vi "Initialization.vi"(8 "error in":errorcluster, 11 "Data Cluster":T1={"Status"="", "Image"=[], "Device Settings"={"ROI"={"_Horizontal"=0, "_Horizontal Width"=0, "_Horizontal Binning"=0, "_Vertical"=0, "_Vertical Width"=0, "_Vertical Binning"=0}, "Gating"={"_GatingMode"=enum."None", "_RepetitiveGate"={"delay"=0.0, "width"=0.0}}, "Readout Control"={"Accumulations"=0}, "AD Conversion"={"AdcSpeed"=0.0, "AdcEMGain"=0, "AdcBitDepth"=0, "AdcAnalogGain"=enum."Low", "AdcQuality"=enum."LowNoise"}, "Intensifier"={"EnableIntensifier"=FALSE, "IntensifierStatus"=enum."None", "IntensifierGain"=0, "_EMIccdGainControlMode"=enum."None", "EMIccdGain"=0, "GatingSpeed"=enum."None"}, "Sensor Temperature"={"SensorTemperatureSetPoint"=0.0, "SensorTemperatureReading"=0.0, "SensorTemperatureStatus"=enum."None"}}, "-Picam Object"=refnum}) -> (0 "error out":errorcluster, 3 "Data Cluster out":T1={"Status"="", "Image"=[], "Device Settings"={"ROI"={"_Horizontal"=0, "_Horizontal Width"=0, "_Horizontal Binning"=0, "_Vertical"=0, "_Vertical Width"=0, "_Vertical Binning"=0}, "Gating"={"_GatingMode"=enum."None", "_RepetitiveGate"={"delay"=0.0, "width"=0.0}}, "Readout Control"={"Accumulations"=0}, "AD Conversion"={"AdcSpeed"=0.0, "AdcEMGain"=0, "AdcBitDepth"=0, "AdcAnalogGain"=enum."Low", "AdcQuality"=enum."LowNoise"}, "Intensifier"={"EnableIntensifier"=FALSE, "IntensifierStatus"=enum."None", "IntensifierGain"=0, "_EMIccdGainControlMode"=enum."None", "EMIccdGain"=0, "GatingSpeed"=enum."None"}, "Sensor Temperature"={"SensorTemperatureSetPoint"=0.0, "SensorTemperatureReading"=0.0, "SensorTemperatureStatus"=enum."None"}}, "-Picam Object"=refnum})   [LabVIEW 2019, in "Camera.lvlib"]
uses:
  Camera.lvlib
  Module Data--cluster.ctl
  Camera-LVClass/Picam_class/Picam.lvclass
  ROI--cluster.ctl
  picam32_LabView_SDK/PICam_lib/types/PicamGatingMode.ctl
  picam32_LabView_SDK/PICam_lib/types/PicamPulse.ctl
  picam32_LabView_SDK/PICam_lib/Ctrls/PicamAdcAnalogGain.ctl
  picam32_LabView_SDK/PICam_lib/Ctrls/PicamAdcQuality.ctl
  picam32_LabView_SDK/PICam_lib/types/PicamIntensifierStatus.ctl
  picam32_LabView_SDK/PICam_lib/types/PicamEMIccdGainControlMode.ctl
  picam32_LabView_SDK/PICam_lib/types/PicamGatingSpeed.ctl
  picam32_LabView_SDK/PICam_lib/types/PicamSensorTemperatureStatus.ctl
  picam32_LabView_SDK/PICam_lib/PICam.lvlib
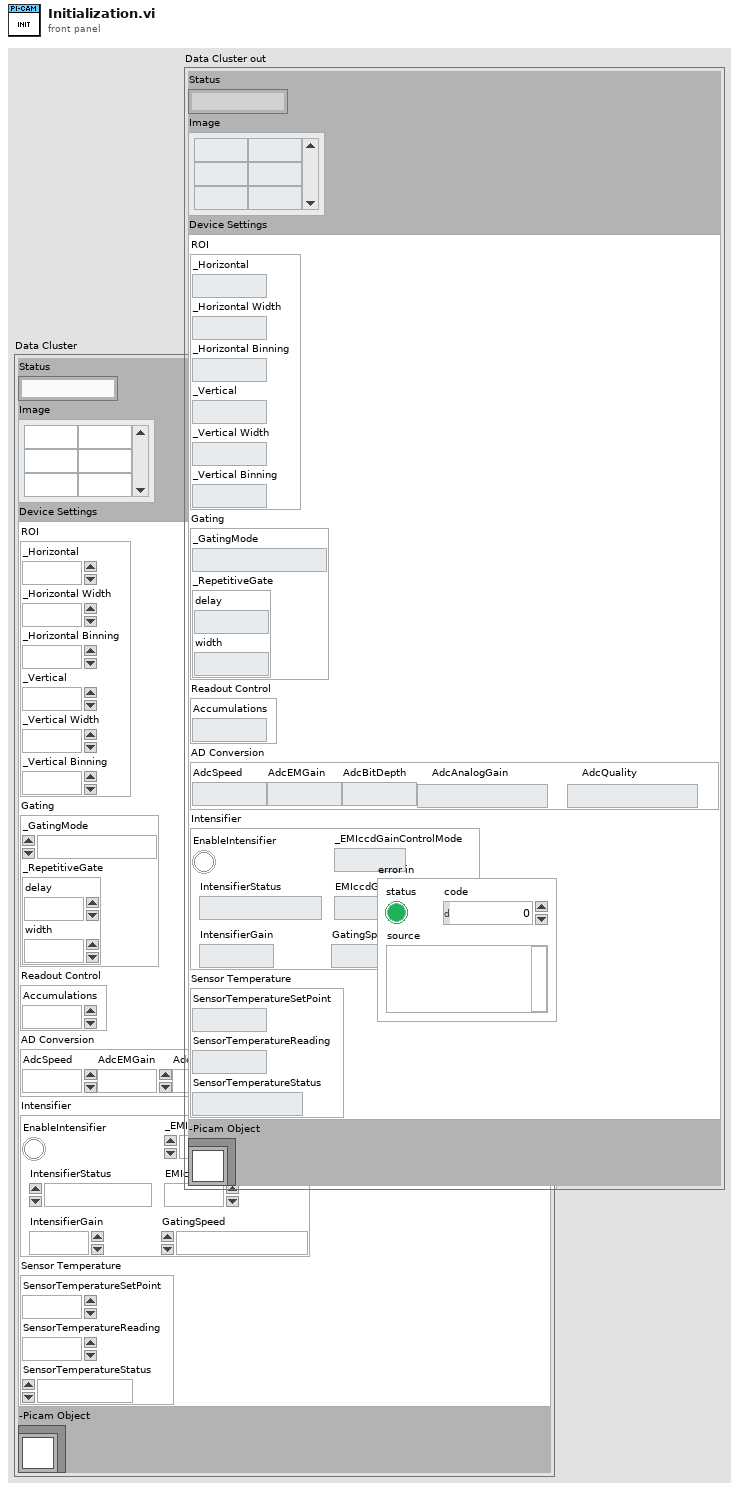
[diagram p1: front panel]
types:
  T1 = typedef "Camera.lvlib/Module Data--cluster.ctl" = cluster{"Status":string, "Image":u16[][], "Device Settings":cluster{"ROI":T2, "Gating":cluster{"_GatingMode":T3, "_RepetitiveGate":T4}, "Readout Control":cluster{"Accumulations":i64}, "AD Conversion":cluster{"AdcSpeed":dbl, "AdcEMGain":i32, "AdcBitDepth":i32, "AdcAnalogGain":T5, "AdcQuality":T6}, "Intensifier":cluster{"EnableIntensifier":bool, "IntensifierStatus":T7, "IntensifierGain":i32, "_EMIccdGainControlMode":T8, "EMIccdGain":i32, "GatingSpeed":T9}, "Sensor Temperature":cluster{"SensorTemperatureSetPoint":dbl, "SensorTemperatureReading":dbl, "SensorTemperatureStatus":T10}}, "-Picam Object":refnum<class "Picam.lvclass">}
  T2 = typedef "Camera.lvlib/ROI--cluster.ctl" = cluster{"_Horizontal":i32, "_Horizontal Width":i32, "_Horizontal Binning":i32, "_Vertical":i32, "_Vertical Width":i32, "_Vertical Binning":i32}
  T3 = typedef "PICam.lvlib/PicamGatingMode.ctl" = enum16{"None", "Repetitive", "Sequential", "Custom", "Disabled"}
  T4 = typedef "PICam.lvlib/PicamPulse.ctl" = cluster{"delay":dbl, "width":dbl}
  T5 = typedef "PICam.lvlib/PicamAdcAnalogGain.ctl" = enum16{"None", "Low", "Medium", "High"}
  T6 = typedef "PICam.lvlib/PicamAdcQuality.ctl" = enum16{"None", "LowNoise", "HighCapacity", "ElectronMultiplied", "HighSpeed"}
  T7 = typedef "PICam.lvlib/PicamIntensifierStatus.ctl" = enum16{"None", "PoweredOff", "PoweredOn"}
  T8 = typedef "PICam.lvlib/PicamEMIccdGainControlMode.ctl" = enum16{"None", "Optimal", "Manual"}
  T9 = typedef "PICam.lvlib/PicamGatingSpeed.ctl" = enum16{"None", "Fast", "Slow"}
  T10 = typedef "PICam.lvlib/PicamSensorTemperatureStatus.ctl" = enum16{"None", "Unlocked", "Locked", "Faulted"}
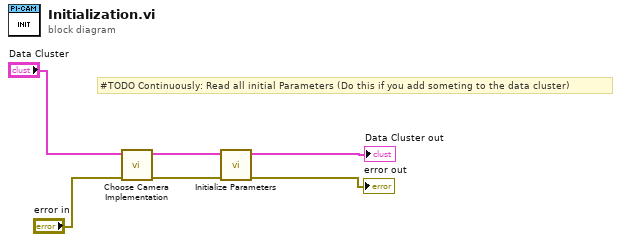
[diagram p0: block diagram]
diagram:
  # "#TODO Continuously: Read all initial Parameters (Do this if you add someting to the data cluster)"
  n1 = call "Choose Camera Implementation.vi"("error in (no error)"="error in", "Data Cluster in"="Data Cluster") -> ("error out"=w1:errorcluster, "Data Cluster out"=w5:T1)  [unwired: 8 in]
  n2 = call "Initialize Parameters.vi"("error in (no error)"=w1, "Data Cluster in"=w5) -> ("error out"=→"error out":errorcluster, "Data Cluster out"=→"Data Cluster out":T1)  [unwired: 8 in]
